vi "Dashboard Cursor Interpolation.vi"(5 "Remove Cursor":bool, 7 "Add Cursor":bool, 8 "Joystick Input":dbl[](array[numeric]), 9 "Graph Detail":i32, 10 "Interpolation Method":i32(ring)=1 items=["nearest", "linear", "spline", "cubic Hermite", "Lagrange"], 11 "Interpolation Points":refnum<vi>) -> (0 "Joystick Output":dbl[](array[numeric]))   [LabVIEW 2018]
uses:
  <vilib>/Utility/miscctls.llb/LVCursorListTypeDef.ctl
  <vilib>/gmath/NI_Gmath.lvlib
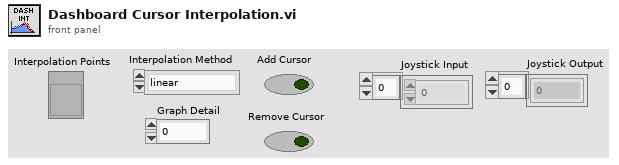
[diagram p1: front panel]
types:
  T1 = typedef "LVCursorListTypeDef.ctl" = cluster{"Name":string, "Color":u32, "Style":u8, "Point Style":u8, "Name Visible":bool, "Allow Drag":bool, "Cursor Mode":u32, "Plot":i32, "Index":i32, "Position":cluster{"X":dbl, "Y":dbl}, "X Scale":u32, "Y Scale":u32, "Watch Plots":i32[], "Watch All Plots":bool, "Plot Area":i32, "Label Offset":cluster{"X":dbl, "Y":dbl}}[]
  T2 = cluster{"Name":string, "Color":u32, "Style":u8, "Point Style":u8, "Name Visible":bool, "Allow Drag":bool, "Cursor Mode":u32, "Plot":i32, "Index":i32, "Position":cluster{"X":dbl, "Y":dbl}, "X Scale":u32, "Y Scale":u32, "Watch Plots":i32[], "Watch All Plots":bool, "Plot Area":i32, "Label Offset":cluster{"X":dbl, "Y":dbl}}
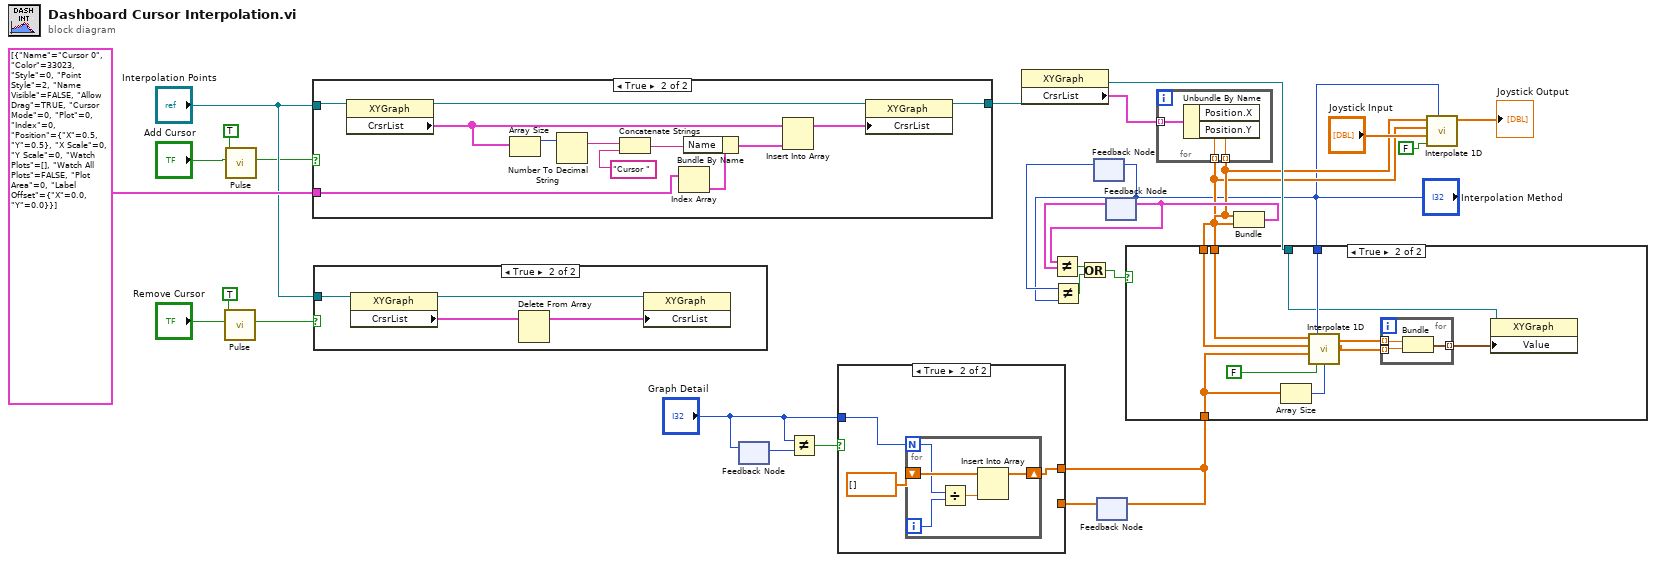
[diagram p0: block diagram]
diagram:
  n1 = call "Pulse.vi"("Input"="Remove Cursor", "Rising Edge?"=TRUE) -> ("Output"=w23:bool)  [unwired: 9 in]
  n2 = call "Pulse.vi"("Input"="Add Cursor", "Rising Edge?"=TRUE) -> ("Output"=w21:bool)  [unwired: 9 in]
  n3 = case shown="True" w21 {
    tunnel: T1 [{"Name"="Cursor 0", "Color"=33023, "Style"=0, "Point Style"=2, "Name Visible"=FALSE, "Allow Drag"=TRUE, "Cursor Mode"=0, "Plot"=0, "Index"=0, "Position"={"X"=0.5, "Y"=0.5}, "X Scale"=0, "Y Scale"=0, "Watch Plots"=[], "Watch All Plots"=FALSE, "Plot Area"=0, "Label Offset"={"X"=0.0, "Y"=0.0}}] ("Cursor List") -> [_ w38]
    tunnel: "Interpolation Points" -> [w29 w33]
    tunnel: [w29 w30] -> w25
    frame False {
    }
    frame True {
      n4 = property class="XYGraph"(reference=w33) -> (reference out=w32:refnum<vi>, "CrsrList"=w34:T1)  [unwired: 1 in, 1 out]
      n5 = Array Size(array=w34) -> (size(s)=w40:i32)
      n6 = Number To Decimal String(number=w40) -> (decimal integer string=w39:string)  [unwired: 1 in]
      n7 = Concatenate Strings("Cursor ", w39) -> (w36:string)
      n8 = Index Array(array=w38) -> (element=w37:T2)  [unwired: 1 in]
      n9 = Bundle By Name(cluster=w37, "Name"=w36) -> (w35:T2)
      n10 = Insert Into Array(array=w34, new element=w35) -> (w31:T1)  [unwired: 1 in]
      n11 = property class="XYGraph"(reference=w32, "CrsrList"=w31) -> (reference out=w30:refnum<vi>)  [unwired: 1 in, 1 out]
    }
  }
  n12 = case shown="True" w23 {
    tunnel: "Interpolation Points" -> [_ w43]
    frame False {
    }
    frame True {
      n13 = property class="XYGraph"(reference=w43) -> (reference out=w42:refnum<vi>, "CrsrList"=w44:T1)  [unwired: 1 in, 1 out]
      n14 = Delete From Array(array=w44) -> (array with subset deleted=w45:T1)  [unwired: 2 in, 1 out]
      n15 = property class="XYGraph"(reference=w42, "CrsrList"=w45) -> ()  [unwired: 1 in, 2 out]
    }
  }
  n16 = feedback-in #1("Graph Detail") -> ()
  n17 = feedback #1() -> (w15:i32)  [unwired: 1 in]
  n18 = Not Equal?(x="Graph Detail", y=w15) -> (x != y?=w16:bool)
  n19 = property class="XYGraph"(reference=w25) -> (reference out=w26:refnum<vi>, "CrsrList"=w13:T1)  [unwired: 1 in, 1 out]
  n20 = feedback-in #2("Interpolation Method") -> ()
  n21 = feedback #2() -> (w7:i32)  [unwired: 1 in]
  n22 = Not Equal?(x=w7, y="Interpolation Method") -> (x != y?=w8:bool)
  n23 = feedback #3() -> (w17:dbl[])  [unwired: 1 in]
  n24 = case shown="True" w16 {
    tunnel: [w46 w49] -> w18
    tunnel: "Graph Detail" -> [_ w48]
    tunnel: w17 -> [w46 _]
    frame False {
    }
    frame True {
      n25 = for {
        N: w48 -> [w51]
        shift-right: [w53] -> w49
        shift-left: dbl[] [] -> [w52]
        i -> [w50]
        n26 = Divide(x=w50, y=w51) -> (x/y=w54:dbl)
        n27 = Insert Into Array(array=w52, new element=w54) -> (w53:dbl[])  [unwired: 1 in]
      }
    }
  }
  n28 = feedback-in #3(w18) -> ()
  n29 = feedback #4() -> (w11:cluster{dbl[], dbl[]})  [unwired: 1 in]
  n30 = for {
    tunnel: w13 -> [w57] mode=indexing
    tunnel: [w56] -> w4 mode=indexing
    tunnel: [w55] -> w5 mode=indexing
    n31 = Unbundle By Name(w57) -> ("Position.X"=w56:dbl, "Position.Y"=w55:dbl)
  }
  n32 = Bundle(w5, w4) -> (w12:cluster{dbl[], dbl[]})  [unwired: 1 in]
  n33 = Not Equal?(x=w12, y=w11) -> (x != y?=w9:bool)
  n34 = Or(x=w9, y=w8) -> (x .or. y?=w10:bool)
  n35 = feedback-in #4(w12) -> ()
  n36 = case shown="True" w10 {
    tunnel: "Interpolation Method" -> [_ w67]
    tunnel: w4 -> [_ w66]
    tunnel: w5 -> [_ w65]
    tunnel: w26 -> [_ w59]
    tunnel: w18 -> [_ w58]
    frame False {
    }
    frame True {
      n37 = Array Size(array=w58) -> (size(s)=w63:i32)
      n38 = call <vilib>:"Interpolate 1D.vi"("ntimes"=w63, "method"=w67, "X is monotonic"=FALSE, "xi"=w58, "X"=w66, "Y"=w65) -> ("xi used"=w61:dbl[], "yi"=w62:dbl[])  [unwired: 3 in, 1 out]
      n39 = for {
        tunnel: w62 -> [w69] mode=indexing
        tunnel: w61 -> [w68] mode=indexing
        tunnel: [w70] -> w60 mode=indexing
        n40 = Bundle("Numeric"=w68, "Numeric"=w69) -> (w70:cluster{"Numeric":dbl, "Numeric":dbl})  [unwired: 1 in]
      }
      n41 = property class="XYGraph"(reference=w59, "Value"=w60) -> ()  [unwired: 1 in, 2 out]
    }
  }
  n42 = call <vilib>:"Interpolate 1D.vi"("method"="Interpolation Method", "X is monotonic"=FALSE, "xi"="Joystick Input", "X"=w4, "Y"=w5) -> ("yi"=→"Joystick Output":dbl[])  [unwired: 4 in, 2 out]
